vi "load config.vi"(8 "error in (no error)":errorcluster, 10 "cfg file name":string="ic_sparc.cfg", 11 "Channel in":refnum<class "Channel.lvclass">) -> (0 "error out":errorcluster, 3 "Channel out":refnum<class "Channel.lvclass">)   [LabVIEW 2018, in "Channel.lvclass"]
uses:
  Channel.lvclass
  Channel.lvclass/Channel.ctl
  Interface/Interface.lvclass/Interface.ctl
  <vilib>/Utility/config.llb/Read Key (String).vi
  Interface/Interface.lvclass
  <vilib>/Utility/config.llb/NI_LVConfig.lvlib
panel:
  out "value 2":T1
  out "#FRAMES":u32
  out "EXPTIME":dbl
  out "JSON string":string
  out "output cluster":T2={"ACQUISITION_MODE"=1, "TRIGGER_MODE"=0, "READ_MODE"=4, "PREAMP"=0, "READOUT_RATE"=0, "VERTICAL_SHIFT_SPEED"=3, "EM_MODE"=0, "EM_GAIN"=2, "SHUTTER_MODE"=2, "SHUTTER_TTL"=0, "SHUTTER_OPENNING_TIME"=50, "SHUTTER_CLOSING_TIME"=50, "VBIN"=1, "HBIN"=1, "INITIAL_LINE"=1, "INITIAL_COLUMN"=1, "FINAL_LINE"=1024, "FINAL_COLUMN"=1024, "FRAME_TRANSFER"=FALSE, "VERTICAL_CLOCK_VOLTAGE"=0, "AD_CHANNEL"=0} {"VERTICAL_CLOCK_VOLTAGE" items=["Normal", "+1", "+2", "+3", "+4"]; "SHUTTER_TTL" items=["TTL Low", "TTl High"]; "SHUTTER_MODE" items=["Fully Auto", "OPEN", "CLOSED"]; "EM_MODE" items=["Electron Multiplying", "Conventional"]; "VERTICAL_SHIFT_SPEED" items=["0.6", "1.13", "2.2", "4.33"]; "READOUT_RATE" items=["1 MHz", "10 MHz", "20 MHz", "30 MHz"]; "PREAMP" items=["Gain 1", "Gain 2"]; "READ_MODE" items=["Full Vertical Binning", "Multi-Track", "Random-track", "Single-Track", "Image"]; "TRIGGER_MODE" items=["Internal", "External", "N/A", "N/A", "N/A", "N/A", "External Start"]; "ACQUISITION_MODE" items=["N/A", "Single", "Accumulate", "Kinetic", "Fast Kinetic"]}
  out "value":string
  out "file created?":bool
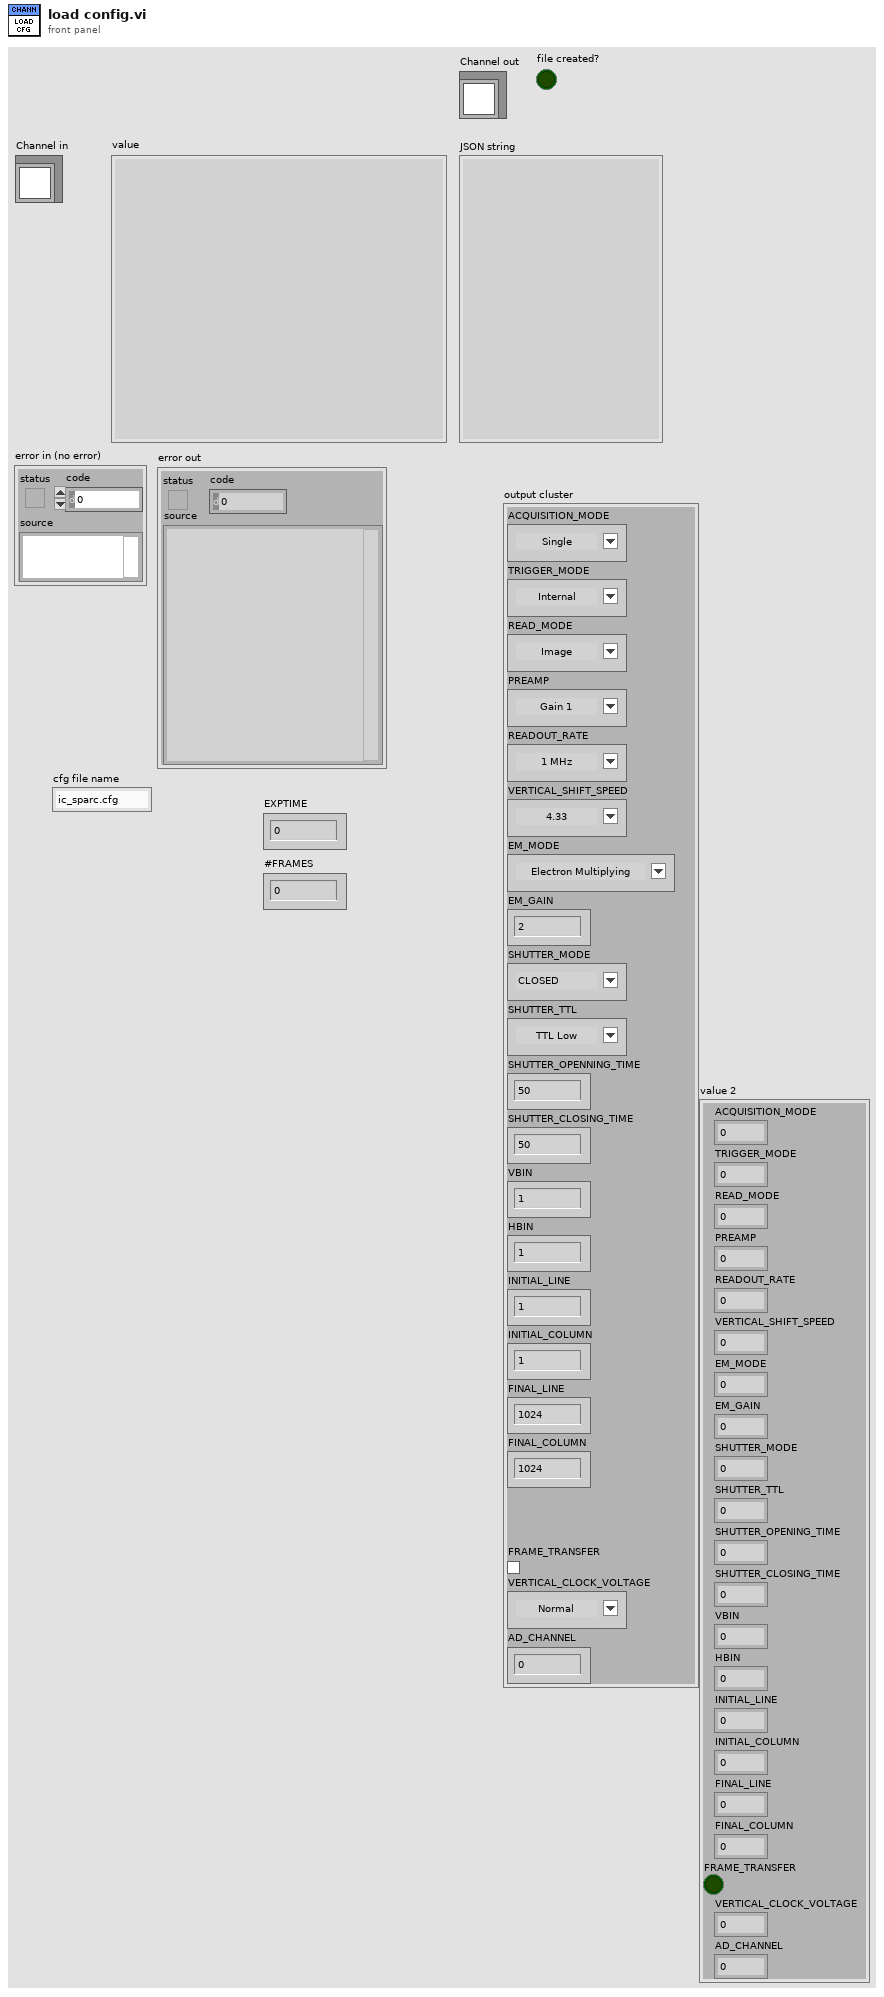
[diagram p1: front panel]
types:
  T1 = cluster{"ACQUISITION_MODE":u8, "TRIGGER_MODE":u8, "READ_MODE":u8, "PREAMP":u8, "READOUT_RATE":u8, "VERTICAL_SHIFT_SPEED":u8, "EM_MODE":u8, "EM_GAIN":u16, "SHUTTER_MODE":u8, "SHUTTER_TTL":u8, "SHUTTER_OPENING_TIME":u16, "SHUTTER_CLOSING_TIME":u16, "VBIN":u16, "HBIN":u16, "INITIAL_LINE":u16, "INITIAL_COLUMN":u16, "FINAL_LINE":u16, "FINAL_COLUMN":u16, "FRAME_TRANSFER":bool, "VERTICAL_CLOCK_VOLTAGE":u8, "AD_CHANNEL":u32}
  T2 = cluster{"ACQUISITION_MODE":u8, "TRIGGER_MODE":u8, "READ_MODE":u8, "PREAMP":u8, "READOUT_RATE":u8, "VERTICAL_SHIFT_SPEED":u8, "EM_MODE":u8, "EM_GAIN":u16, "SHUTTER_MODE":u8, "SHUTTER_TTL":u8, "SHUTTER_OPENNING_TIME":u16, "SHUTTER_CLOSING_TIME":u16, "VBIN":u16, "HBIN":u16, "INITIAL_LINE":u16, "INITIAL_COLUMN":u16, "FINAL_LINE":u16, "FINAL_COLUMN":u16, "FRAME_TRANSFER":bool, "VERTICAL_CLOCK_VOLTAGE":u8, "AD_CHANNEL":u32}
  T3 = typedef "NI_LVConfig.lvlib/Config Data RefNum.ctl" = refnum<k1>
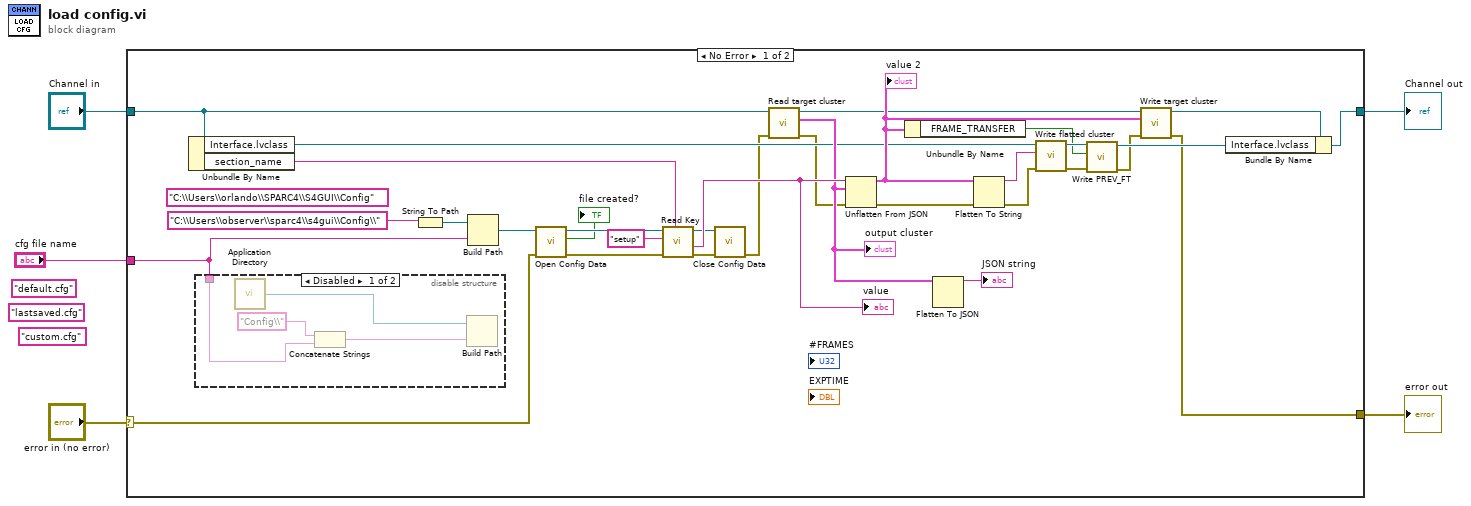
[diagram p0: block diagram]
diagram:
  (unwired) "custom.cfg" ("name or relative path")
  (unwired) "lastsaved.cfg" ("name or relative path")
  (unwired) "default.cfg" ("name or relative path")
  n1 = case shown="No Error" "error in (no error)" {
    selector: "error in (no error)" -> [w32 w43]
    tunnel: [w9 w43] -> w4
    tunnel: [w33 w42] -> w2
    tunnel: "Channel in" -> [w19 w42]
    tunnel: "cfg file name" -> [w8 _]
    frame No Error {
      (unwired) "C:\\Users\\orlando\\SPARC4\\S4GUI\\Config"
      n2 = Unbundle By Name(w19) -> ("Interface.lvclass"=w14:refnum<class "Interface.lvclass">, "section_name"=w36:string)
      n3 = disable-structure shown="Disabled" {
        disable-tunnel: w8 -> [w38 _]
        frame Disabled {
          n4 = call <vilib>:"Application Directory.vi"() -> ("Application Directory"=w40:path)
          n5 = Concatenate Strings("Config\\" ("string"), w38) -> (w39:string)
          n6 = Build Path(base path=w40, name or relative path=w39) -> ()  [unwired: 1 out]
        }
        frame Enabled {
        }
      }
      n7 = String To Path(string="C:\\Users\\observer\\sparc4\\s4gui\\Config\\") -> (path=w7:path)
      n8 = Build Path(base path=w7, name or relative path=w8) -> (appended path=w37:path)
      n9 = call <vilib>:"Open Config Data.vi"("error in (no error)"=w32, "configuration file path"=w37) -> ("error out"=w28:errorcluster, "file created?"=→"file created?":bool, "refnum"=w35:T3)  [unwired: 7 in]
      n10 = call-poly <vilib>:"Read Key.vi"("section"=w36, "error in (no error)"=w28, "key"="setup", "refnum"=w35) -> ("error out"=w24:errorcluster, "value"=w29:string, "refnum out"=w25:T3)  [unwired: 4 in, 1 out]
      "value" <- w29
      n11 = call <vilib>:"Close Config Data.vi"("error in (no error)"=w24, "refnum"=w25) -> ("error out"=w12:errorcluster)  [unwired: 8 in, 1 out]
      n12 = call-dynamic "Read target cluster.vi"("error in (no error)"=w12, "Channel in"=w19) -> ("error out"=w11:errorcluster, "target cluster"=w17:T1, "Channel out"=w15:refnum<class "Channel.lvclass">)  [unwired: 7 in]
      "output cluster" <- w17
      n13 = Unflatten From JSON(JSON string=w29, type and defaults=w17, error in (no error)=w11) -> (value=w16:T1, error out=w13:errorcluster)  [unwired: 4 in]
      "value 2" <- w16
      n14 = Unbundle By Name(w16) -> ("FRAME_TRANSFER"=w20:bool)
      n15 = Flatten To JSON(anything=w17) -> (JSON string=→"JSON string":string)  [unwired: 2 in, 1 out]
      n16 = Flatten To String(anything=w16, error in (no error)=w13) -> (data string=w31:string, error out=w30:errorcluster)  [unwired: 2 in, 1 out]
      n17 = call "Write flatted cluster.vi"("error in (no error)"=w30, "flatted cluster"=w31, "Interface in"=w14) -> ("error out"=w22:errorcluster, "Interface out"=w23:refnum<class "Interface.lvclass">)  [unwired: 7 in]
      n18 = call-dynamic "Write PREV_FT.vi"("error in (no error)"=w22, "PREV_FT"=w20, "Interface in"=w23) -> ("error out"=w10:errorcluster, "Interface out"=w21:refnum<class "Interface.lvclass">)  [unwired: 7 in]
      n19 = call-dynamic "Write target cluster.vi"("error in (no error)"=w10, "target cluster"=w16, "Channel in"=w15) -> ("error out"=w9:errorcluster, "Channel out"=w18:refnum<class "Channel.lvclass">)  [unwired: 7 in]
      n20 = Bundle By Name(cluster=w18, "Interface.lvclass"=w21) -> (w33:refnum<class "Channel.lvclass">)
    }
    frame Error {
    }
  }
  "error out" <- w4
  "Channel out" <- w2
